vi "com发送.vi"(8 "发送数据":string, 10 "RS232波特率":T1(ring), 11 "RS232端口":refnum<visa-resource-name>="COM1") -> ()   [LabVIEW 2010]
uses:
  <vilib>/Instr/_visa.llb/VISA Configure Serial Port (Instr).vi
panel:
  in  "数据长度":u16
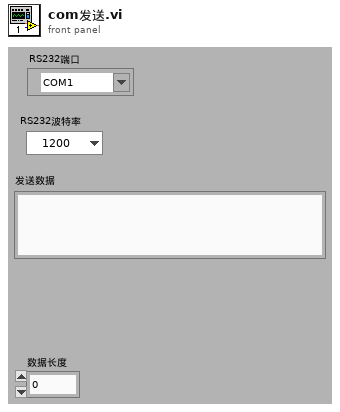
[diagram p1: front panel]
types:
  T1 = enum16{"1200", "2400", "4800", "9600", "19200", "57600", "115200", ""}
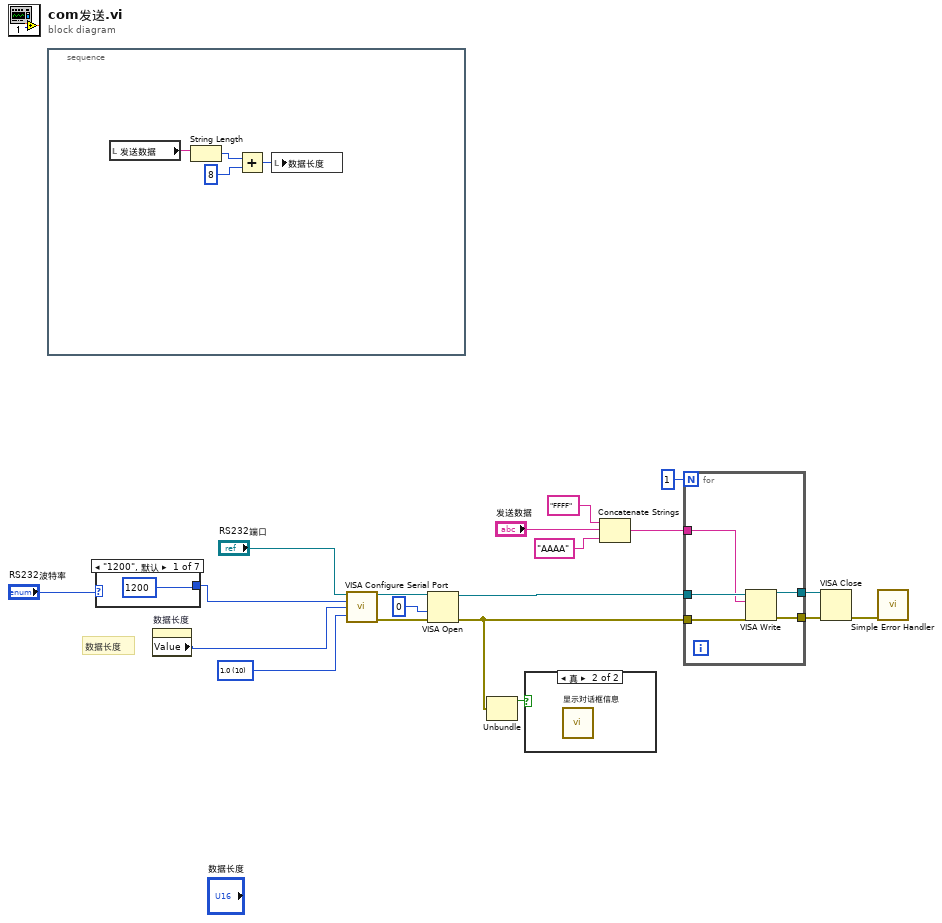
[diagram p0: block diagram]
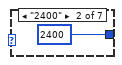
[diagram p2: hidden frame]
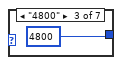
[diagram p3: hidden frame]
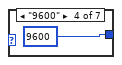
[diagram p4: hidden frame]
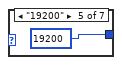
[diagram p5: hidden frame]
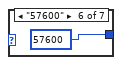
[diagram p6: hidden frame]
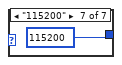
[diagram p7: hidden frame]
diagram:
  w10 = u16 10 items=["1.0"=10, "1.5"=15, "2.0"=20] ("stop bits (10: 1 bit)")
  # "数据长度"
  n1 = stacked-sequence {
    frame #0 {
      n2 = local read "发送数据"() -> (w23:string)
      n3 = String Length(string=w23) -> (length=w22:i32)
      n4 = Add(x=w22, y=8) -> (x+y=w20:i32)
      n5 = local write "数据长度"(w20) -> ()
    }
  }
  n6 = case shown="\"1200\", 默认" "RS232波特率" {
    tunnel: [u32 1200 u32 2400 u32 4800 u32 9600 u32 19200 u32 57600 u32 115200] -> w6
    frame "1200", Default {
    }
    frame "2400" {
    }
    frame "4800" {
    }
    frame "9600" {
    }
    frame "19200" {
    }
    frame "57600" {
    }
    frame "115200" {
    }
  }
  n7 = property on="数据长度" class="DigNum (严格)"() -> ("Value"=w8:u16)  [unwired: 2 in, 2 out]
  n8 = call-poly "VISA Configure Serial Port"("VISA resource name"="RS232端口", "baud rate (9600)"=w6, "data bits (8)"=w8, "stop bits (10: 1 bit)"=w10) -> ("VISA resource name out"=w16:refnum<visa-resource-name>, "error out"=w12:errorcluster)  [unwired: 10 in]
  n9 = VISA Open(access mode=u32 0, error in (no error)=w12, VISA resource name=w16) -> (VISA resource name=w15:refnum<visa-resource-name>, error out=w9:errorcluster)  [unwired: 2 in]
  n10 = Unbundle(w9) -> ("status"=w11:bool)  [unwired: 2 out]
  n11 = case shown="真" w11 {
    frame False {
    }
    frame True {
      n12 = call "显示对话框信息"() -> ()  [unwired: 10 in, 2 out]
    }
  }
  n13 = Concatenate Strings("FFFF" ("字符串"), "发送数据", "AAAA" ("字符串")) -> (w2:string)
  n14 = for {
    N: 1 -> [_]
    tunnel: [w35] -> w19
    tunnel: [w34] -> w18
    tunnel: w15 -> [w33]
    tunnel: w9 -> [w32]
    tunnel: w2 -> [w31]
    n15 = VISA Write(VISA resource name=w33, write buffer=w31, error in (no error)=w32) -> (VISA resource name out=w35:refnum<visa-resource-name>, error out=w34:errorcluster)  [unwired: 1 out]
  }
  n16 = VISA Close(VISA resource name=w19, error in (no error)=w18) -> (error out=w17:errorcluster)
  n17 = call <vilib>:"Simple Error Handler.vi"("error in (no error)"=w17) -> ()  [unwired: 4 in, 5 out]
